vi "Template UE+DVR.vi"() -> ()   [LabVIEW 2017]
uses:
  Error Handler/Controls/Error Message.ctl
  Error Handler/Controls/Error Level.ctl
  Controller/Controls/CNTRLR - Message.ctl
  Controller/Controls/CNTRLR - Command.ctl
  Configuration/Controls/Database Message.ctl
  Configuration/Controls/Database Command.ctl
  Configuration/Controls/Database Overhead.ctl
  Configuration/Controls/Database Status.ctl
  Configuration/Controls/Database Record.ctl
panel:
  in  "DB Overhead DVR":refnum<data-value>
  in  "DB Message":refnum<user-event>
  in  "CNTRLR to UI":refnum<queue>
  in  "Stop DVR":refnum<data-value>
  in  "Stop":refnum<user-event>
  in  "Error Message":refnum<user-event>
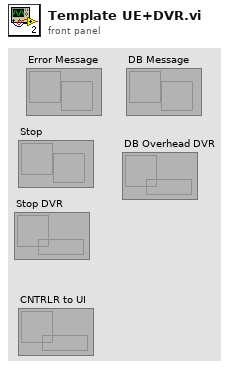
[diagram p1: front panel]
types:
  T1 = typedef "Database Overhead.ctl" = cluster{"DB Status":T2, "DB Records":T3[]}
  T2 = typedef "Database Status.ctl" = enum16{"Unlocked", "Locked"}
  T3 = typedef "Database Record.ctl" = cluster{"Wash Step":string, "Station":string, "Step Duration":u32}
  T4 = typedef "Database Message.ctl" = cluster{"DB Command":T5, "DB Data":variant}
  T5 = typedef "Database Command.ctl" = enum16{"Read Records", "Query Timing", "Insert New Data", "Update Data"}
  T6 = typedef "CNTRLR - Message.ctl" = cluster{"CMD":T7, "Data":variant}
  T7 = typedef "CNTRLR - Command.ctl" = enum16{"Idle", "Stop", "Error"}
  T8 = typedef "Error Message.ctl" = cluster{"Error Level":T9, "Error Data":variant}
  T9 = typedef "Error Level.ctl" = enum16{"Minor Error", "Wash Cycle Error", "System Error"}
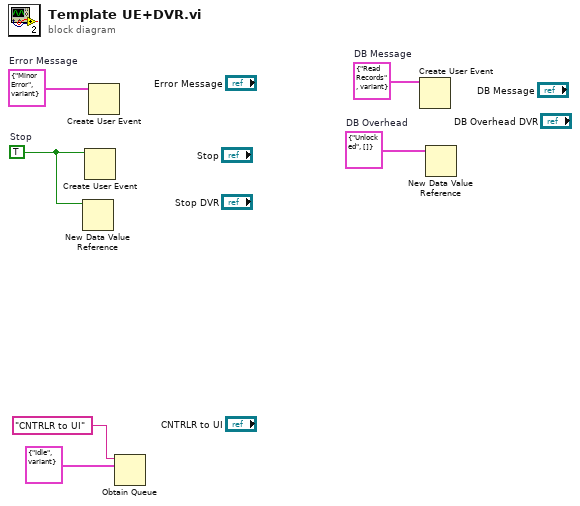
[diagram p0: block diagram]
diagram:
  w1 = T1 {"DB Status"=enum."Unlocked", "DB Records"=[]}  # DB Overhead
  w2 = T4 {"DB Command"=enum."Read Records", "DB Data"=variant}  # DB Message
  w5 = TRUE  # Stop
  w6 = T8 {"Error Level"=enum."Minor Error", "Error Data"=variant}  # Error Message
  n1 = New Data Value Reference(data value=w5) -> ()  [unwired: 1 in, 2 out]
  n2 = Create User Event(user event datatype=w5) -> ()  [unwired: 1 in, 2 out]
  n3 = Create User Event(user event datatype=w6) -> ()  [unwired: 1 in, 2 out]
  n4 = Obtain Queue(name (unnamed)="CNTRLR to UI", element data type=T6 {"CMD"=enum."Idle", "Data"=variant} ("Message")) -> ()  [unwired: 3 in, 3 out]
  n5 = Create User Event(user event datatype=w2) -> ()  [unwired: 1 in, 2 out]
  n6 = New Data Value Reference(data value=w1) -> ()  [unwired: 1 in, 2 out]
